vi "Get Target dt.vi"(11 "Analog Waveform Array in":waveform(dbl)[](array[waveform])) -> (3 "Target dt":dbl)   [LabVIEW 2018, in "Waveform Equalizer.lvlib"]
uses:
  Waveform Equalizer.lvlib
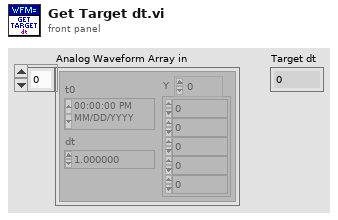
[diagram p1: front panel]
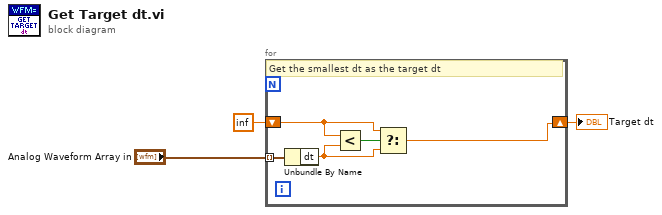
[diagram p0: block diagram]
diagram:
  n1 = for {
    tunnel: "Analog Waveform Array in" -> [w8] mode=indexing
    shift-right: [w4] -> w3
    shift-left: inf -> [w6]
    # "Get the smallest dt as the target dt"
    n2 = Unbundle By Name(w8) -> ("dt"=w5:dbl)
    n3 = Less?(x=w6, y=w5) -> (x < y?=w7:bool)
    n4 = Select(t=w6, s=w7, f=w5) -> (s? t:f=w4:dbl)
  }
  "Target dt" <- w3
